vi "CC Rd Wr Dither Map.vi"(8 "error in (no error)":errorcluster, 10 "Write? (F:Read)":bool, 11 "Dither Map":map{string, T1}(c390)) -> (0 "error out":errorcluster, 3 "Dither Map":map{string, T1}(c390))   [LabVIEW 2021]
uses:
  typedefs/CC Dithering Map.ctl
  typedefs/CC Dithering.ctl
  typedefs/CC cluster Offset Dithering.ctl
  typedefs/CC Dithering Offsets.ctl
  typedefs/CC enum Dithering Types.ctl
  typedefs/CC cluster Random Dithering.ctl
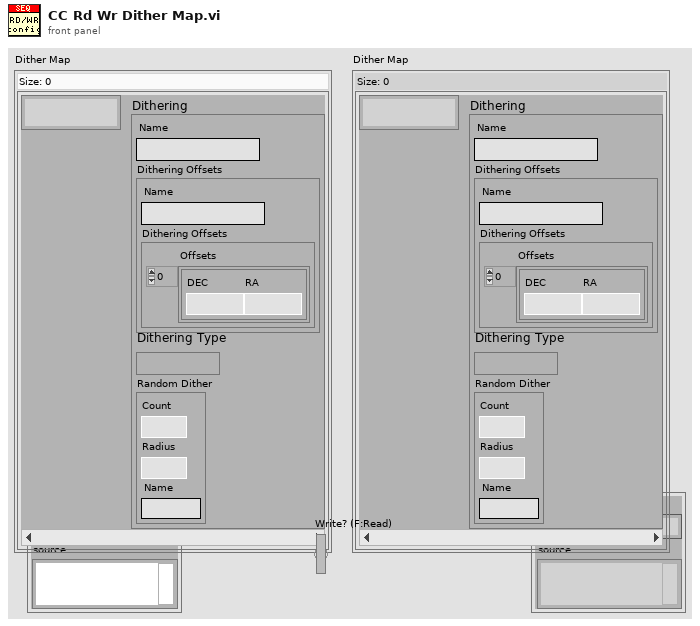
[diagram p1: front panel]
types:
  T1 = typedef "CC Dithering Map.ctl" = cluster{"Name":string, "Dithering Offsets":T2, "Dithering Type":T5, "Random Dither":T6}
  T2 = typedef "CC Dithering.ctl" = cluster{"Name":string, "Dithering Offsets":T3}
  T3 = typedef "CC cluster Offset Dithering.ctl" = cluster{"Offsets":T4[]}
  T4 = typedef "CC Dithering Offsets.ctl" = cluster{"DEC":dbl, "RA":dbl}
  T5 = typedef "CC enum Dithering Types.ctl" = enum16{"Random", "Offsets", "None"}
  T6 = typedef "CC cluster Random Dithering.ctl" = cluster{"Count":i32, "Radius":dbl, "Name":string}
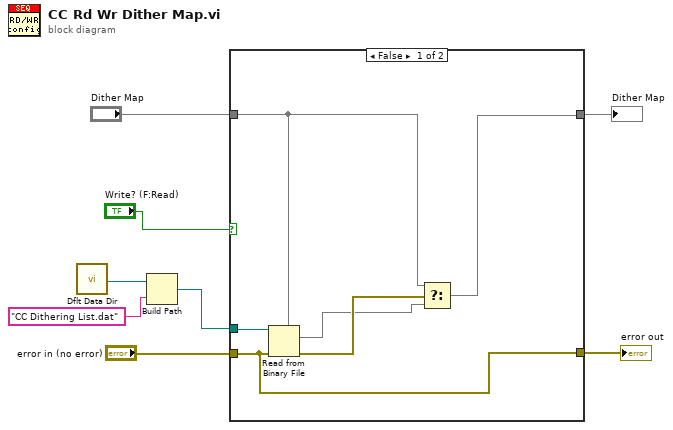
[diagram p0: block diagram]
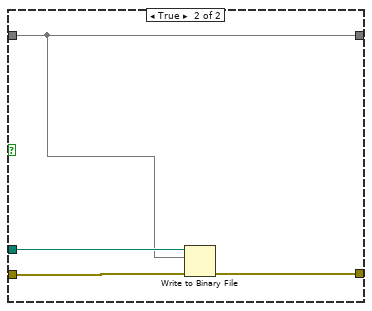
[diagram p2: hidden frame]
diagram:
  n1 = call <vilib>:"Dflt Data Dir.vi"() -> ("App:Default Data Directory"=w5:path)
  n2 = Build Path(base path=w5, name or relative path="CC Dithering List.dat") -> (appended path=w4:path)
  n3 = case shown="False" "Write? (F:Read)" {
    tunnel: "error in (no error)" -> [w12 w16]
    tunnel: "Dither Map" -> [w11 w17]
    tunnel: w4 -> [w14 w18]
    tunnel: [w12 w15] -> w3
    tunnel: [w13 w17] -> w2
    frame False {
      n4 = Read from Binary File(5:w11, 8:w12, 11:w14) -> (0:w10:errorcluster, 2:w9:map{string, T1})  [unwired: 3 in, 2 out]
      n5 = Select(t=w11, s=w10, f=w9) -> (s? t:f=w13:map{string, T1})
    }
    frame True {
      n6 = Write to Binary File(file (use dialog)=w18, data=w17, error in=w16) -> (error out=w15:errorcluster)  [unwired: 3 in, 2 out]
    }
  }
  "error out" <- w3
  "Dither Map" <- w2
